vi "SQL_CountersMonitorUpdate.vi"(8 "Counters Monitor Array":T1(array[cluster]), 9 "SubAssembly":string, 10 "LineName":string, 11 "ConnectionDSN":string) -> ()   [LabVIEW 2017]
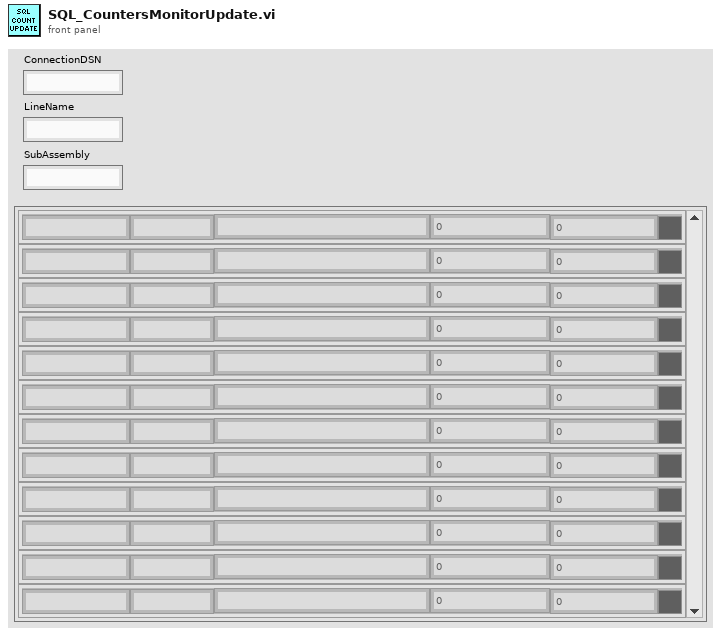
[diagram p1: front panel]
types:
  T1 = cluster{"MachineName":string, "ComponentName":string, "StoppageAlarmCounter":i32, "CurrentCount":i32, "StatusColorBox":u32, "ToolCribPartNumber":string}[]
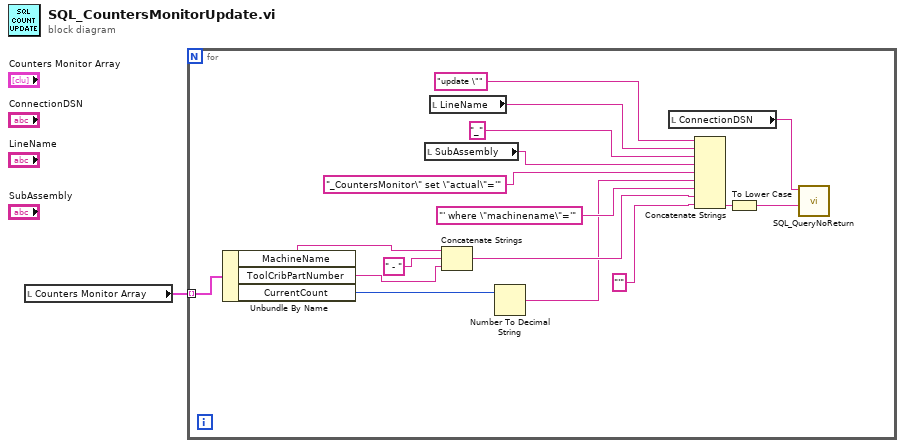
[diagram p0: block diagram]
diagram:
  n1 = local read "Counters Monitor Array"() -> (w1:T1)
  n2 = for {
    tunnel: w1 -> [w18] mode=indexing
    n3 = Unbundle By Name(w18) -> ("MachineName"=w16:string, "ToolCribPartNumber"=w14:string, "CurrentCount"=w3:i32)
    n4 = local read "SubAssembly"() -> (w8:string)
    n5 = local read "LineName"() -> (w10:string)
    n6 = Concatenate Strings(w16, " - ", w14) -> (w5:string)
    n7 = Number To Decimal String(number=w3) -> (decimal integer string=w4:string)  [unwired: 1 in]
    n8 = local read "ConnectionDSN"() -> (w12:string)
    n9 = Concatenate Strings("update \"", w10, "_", w8, "_CountersMonitor\" set \"actual\"='", w4, "' where \"machinename\"='", w5, "'") -> (w17:string)
    n10 = To Lower Case(string=w17) -> (all lower case string=w13:string)
    n11 = call "SQL_QueryNoReturn.vi"("SQL query"=w13, "ConnectionDSN"=w12) -> ()  [unwired: 10 in]
  }
